vi "Read SelfQueue.vi"(8 "error in (no error)":errorcluster, 11 "Execute":refnum<class "Execute.lvclass">) -> (0 "error out":errorcluster, 2 "SelfQueue":refnum<queue>, 3 "Execute":refnum<class "Execute.lvclass">)   [LabVIEW 2018, in "QMH_Class.lvlib" / "TestManager.lvlib" / "Execute.lvclass"]
uses:
  Execute.lvclass
  Message_class/InterfaceMessage/Interface Message.lvclass
  Execute.lvclass/Execute.ctl
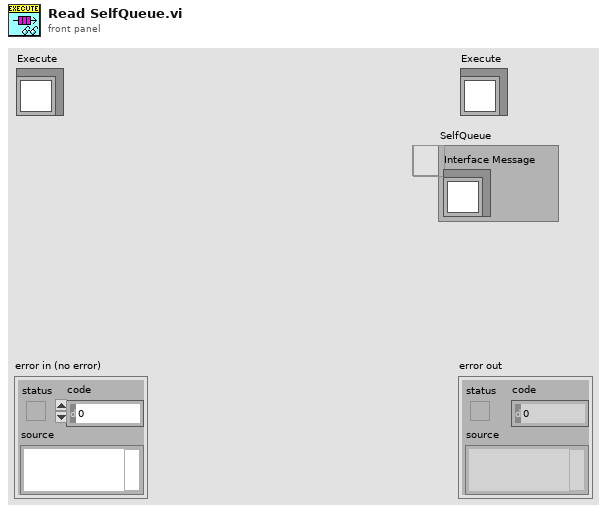
[diagram p1: front panel]
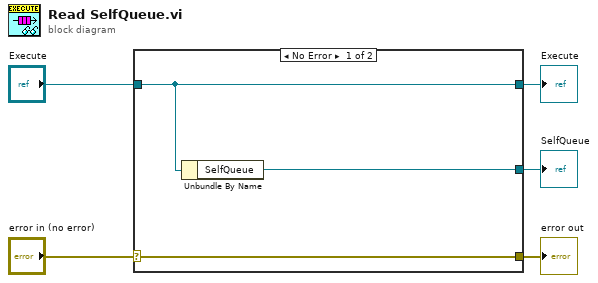
[diagram p0: block diagram]
diagram:
  n1 = case shown="No Error" "error in (no error)" {
    selector: "error in (no error)" -> [w8 w9]
    tunnel: [w8 w9] -> w4
    tunnel: [w7 w10] -> w2
    tunnel: "Execute" -> [w7 w10]
    tunnel: [w6 _] -> w1
    frame No Error {
      n2 = Unbundle By Name(w7) -> ("SelfQueue"=w6:refnum<queue>)
    }
    frame Error {
    }
  }
  "error out" <- w4
  "Execute" <- w2
  "SelfQueue" <- w1
